vi "shutdown.vi"(0 "LINX Resource":T1, 1 "I2C channel wire":u8, 2 "BH1750 address wire":u8, 3 "led output pin":i32) -> ()   [LabVIEW 2021]
uses:
  <vilib>/MakerHub/LINX/Private/Type Defs/LINX Ref.ctl
  <vilib>/MakerHub/LINX/Private/Type Defs/Platform.ctl
  <vilib>/MakerHub/LINX/Private/Type Defs/Interface.ctl
  <vilib>/MakerHub/LINX/Private/Device/Type Defs/LINX Device Config.ctl
  <vilib>/MakerHub/LINX/Private/Device/Type Defs/TCP Config.ctl
  <vilib>/MakerHub/LINX/Private/Device/Type Defs/Channels.ctl
  <vilib>/MakerHub/LINX/Public/Peripherals/Digital/Digital Write 1 Chan.vi
  <vilib>/MakerHub/LINX/Public/Peripherals/Digital/Digital Write N Chans.vi
  <vilib>/MakerHub/LINX/Private/Local IO/LinxDigitalWrite.vi
  <vilib>/MakerHub/LINX/Public/Utilities/Check Channel.vi
  <vilib>/MakerHub/LINX/Private/Utilties/Generate Error.vi
  <vilib>/MakerHub/LINX/LMH-LINX.lvlib
  <vilib>/MakerHub/LINX/Private/Device/Device.lvlib
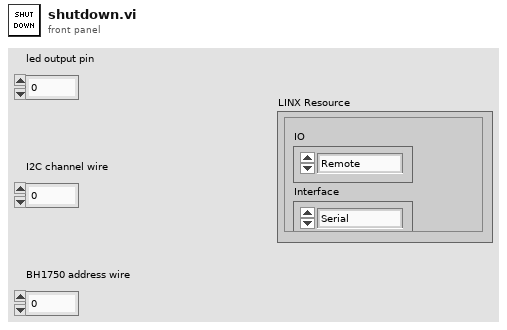
[diagram p1: front panel]
types:
  T1 = typedef "LMH-LINX.lvlib/LINX Ref.ctl" = cluster{"IO":T2, "Interface":T3, "LINX Device Config":T4}
  T2 = typedef "LMH-LINX.lvlib/Platform.ctl" = enum16{"Remote", "Local"}
  T3 = typedef "LMH-LINX.lvlib/Interface.ctl" = enum16{"Serial", "TCP"}
  T4 = typedef "LMH-LINX.lvlib/Device.lvlib/LINX Device Config.ctl" = cluster{"Interface":T3, "COM Port":refnum<visa-resource-name>, "TCP Configuration":T5, "Device Family":u8, "Device ID":u8, "Device Name":string, "TCP Ref":refnum<k5>, "Channels":T6}
  T5 = typedef "LMH-LINX.lvlib/Device.lvlib/TCP Config.ctl" = cluster{"IP Address":string, "Port":u16}
  T6 = typedef "LMH-LINX.lvlib/Channels.ctl" = cluster{"DI":u8[], "DO":u8[], "AI":u8[], "AO":u8[], "PWM":u8[], "QE":u8[], "UART":u8[], "I2C 2":u8[], "SPI":u8[], "CAN":u8[], "Servo":u8[], "AI Ref (V)":dbl, "AI Resolution (Bits)":u8, "AO Ref (V)":dbl, "AO Resolution (Bits)":u8}
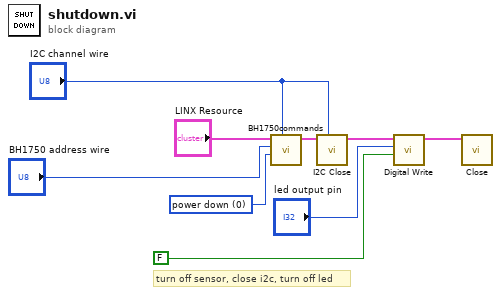
[diagram p0: block diagram]
diagram:
  w6 = u16 0 items=["power down", "Power on", "Reset", "Continuously H- res", "Continuously H- res mode 2", "Continuously L- res", "One time H- res ", "One time H- res mode 2", "One time L res ", "Change Measurement time High bit", "Change Measurement time  Low Bit"] ("Command")
  # "turn off sensor, close i2c, turn off led"
  n1 = call "BH1750commands.vi"("I2C Channel"="I2C channel wire", "Command"=w6, "I2C Slave Address (0)"="BH1750 address wire", "LINX Resource"="LINX Resource") -> ("LINX Resource out"=w7:T1)  [unwired: 5 in, 2 out]
  n2 = call <vilib>:"I2C Close.vi"("I2C Channel (0)"="I2C channel wire", "LINX Resource"=w7) -> ("LINX Resource"=w8:T1)  [unwired: 8 in, 1 out]
  n3 = call-poly <vilib>:"Digital Write.vi"("Output Value"=FALSE, "DO Channel"="led output pin", "LINX Resource"=w8) -> ("LINX Resource"=w4:T1)  [unwired: 7 in, 1 out]
  n4 = call <vilib>:"Close.vi"("LINX Resource"=w4) -> ()  [unwired: 10 in, 1 out]
